vi "PW3337_TEST.vi"() -> ()   [LabVIEW 2017]
panel:
  out "Measurement out":dbl[](array[numeric])
  in  "停止":bool
  out "读取缓冲区":string
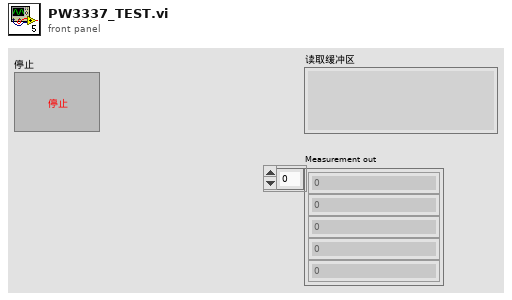
[diagram p1: front panel]
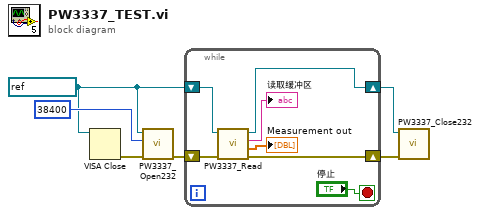
[diagram p0: block diagram]
diagram:
  w3 = refnum<visa-resource-name> "COM14" ("VISA resource name")
  n1 = VISA Close(VISA resource name=w3) -> (error out=w2:errorcluster)  [unwired: 1 in]
  n2 = call "PW3337_Open232.vi"("error in (no error)"=w2, "baud rate (9600)"=u32 38400, "VISA resource name"=w3) -> ("error out"=w5:errorcluster)  [unwired: 7 in, 1 out]
  n3 = while {
    shift-right: [w12] -> w4
    shift-left: w5 -> [w13]
    shift-right: [w9] -> w1
    shift-left: w3 -> [w11]
    stop <- "停止" stop-if-true
    n4 = call "PW3337_Read.vi"("error in (no error)"=w13, "VISA resource name"=w11) -> ("error out"=w12:errorcluster, "Measurement out"=→"Measurement out":dbl[], "读取缓冲区"=→"读取缓冲区":string, "VISA资源名称输出"=w9:refnum<visa-resource-name>)  [unwired: 6 in]
  }
  n5 = call "PW3337_Close232.vi"("error in (no error)"=w4, "VISA resource name"=w1) -> ()  [unwired: 9 in, 1 out]
